vi "例3.7.vi"() -> ()   [LabVIEW 2017]
panel:
  out "最终路径":path
  out "拆分的路径":path
  out "当前VI的路径":path
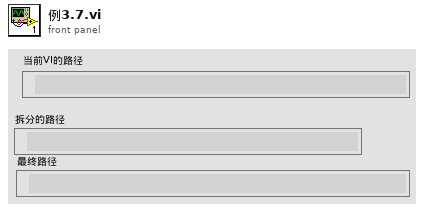
[diagram p1: front panel]
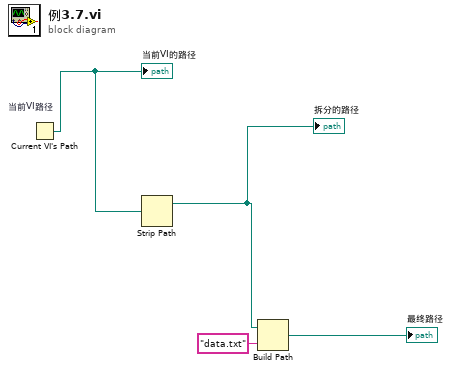
[diagram p0: block diagram]
diagram:
  n1 = Current VI's Path "当前VI路径"() -> (path=w4:path)
  "当前VI的路径" <- w4
  n2 = Strip Path(path=w4) -> (stripped path=w3:path)  [unwired: 1 out]
  "拆分的路径" <- w3
  n3 = Build Path(base path=w3, name or relative path="data.txt" ("名称或相对路径")) -> (appended path=→"最终路径":path)
